vi "GetType.vi"(8 "error in (no error)":errorcluster, 11 "Auto Mute Msg in":refnum<class "Auto Mute Msg.lvclass">) -> (0 "error out":errorcluster, 2 "Data Sample":variant, 3 "Auto Mute Msg out":refnum<class "Auto Mute Msg.lvclass">)   [LabVIEW 2014, in "KIT-QVA.lvlib" / "Auto Mute Msg.lvclass"]
doc: "This VI delivers a sample of the data type format the message expects."
uses:
  Auto Mute Msg.lvclass
  Auto Mute Msg.lvclass/Auto Mute Msg.ctl
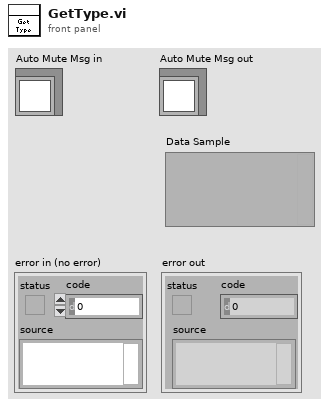
[diagram p1: front panel]
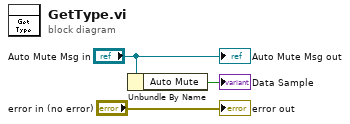
[diagram p0: block diagram]
diagram:
  n1 = Unbundle By Name("Auto Mute Msg in") -> ("Auto Mute"=→"Data Sample":bool)
  "error out" <- "error in (no error)"
  "Auto Mute Msg out" <- "Auto Mute Msg in"
